vi "Untitled 17 (SubVI).vi"(6 "Comp. Eff":dbl, 8 "gammaair":dbl, 9 "Compressor inlet Tempreture (K)":dbl, 10 "Compressor Inlet Pressure (bar)":dbl, 11 "Compressor pressure ratio":dbl) -> (2 "Compressor outlet Temp. (K)":dbl, 3 "Compressor outlet Prs. (bar)":dbl)   [LabVIEW 2019]
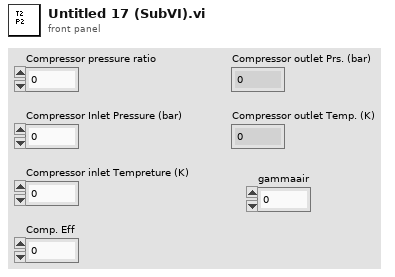
[diagram p1: front panel]
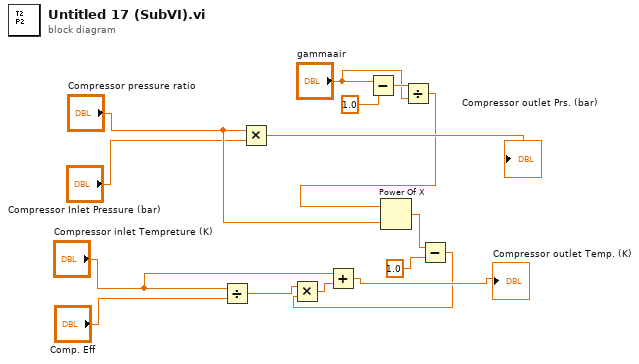
[diagram p0: block diagram]
diagram:
  n1 = Divide(x="Compressor inlet Tempreture (K)", y="Comp. Eff") -> (x/y=w8:dbl)
  n2 = Multiply(x="Compressor pressure ratio", y="Compressor Inlet Pressure (bar)") -> (x*y=→"Compressor outlet Prs. (bar)":dbl)
  n3 = Subtract(x="gammaair", y=1.0) -> (x-y=w3:dbl)
  n4 = Divide(x=w3, y="gammaair") -> (x/y=w1:dbl)
  n5 = Power Of X(1:"Compressor pressure ratio", 2:w1) -> (0:w15:dbl)
  n6 = Subtract(x=w15, y=1.0) -> (x-y=w9:dbl)
  n7 = Multiply(x=w8, y=w9) -> (x*y=w10:dbl)
  n8 = Add(x="Compressor inlet Tempreture (K)", y=w10) -> (x+y=→"Compressor outlet Temp. (K)":dbl)
